vi "Scratchpad.vi"   [LabVIEW 2013]
uses:
  Classes/OSSP_Problem.lvclass
  Classes/GA.lvclass
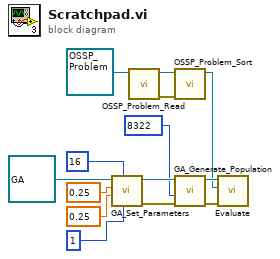
[diagram p0: block diagram]
diagram:
  n1 = call "GA_Set_Parameters.vi"("Population Size"=u8 1, "Dimension"=16, "Control 1Mutation Probability"=0.25, "Crossover Probability"=0.25, "GA in"=refnum<class "GA.lvclass"> refnum ("GA.lvclass")) -> ("error out"=w9:errorcluster, "GA out"=w10:refnum<class "GA.lvclass">)  [unwired: 5 in]
  n2 = call "OSSP_Problem_Read.vi"("OSSP_Problem.lvclass In"=refnum<class "OSSP_Problem.lvclass"> refnum ("OSSP_Problem.lvclass")) -> ("error out"=w12:errorcluster, "OSSP_Problem.lvclass Out"=w13:refnum<class "OSSP_Problem.lvclass">)  [unwired: 9 in]
  n3 = call "OSSP_Problem_Sort.vi"("error in (no error)"=w12, "OSSP_Problem.lvclass In"=w13) -> ("OSSP_Problem.lvclass Out"=w2:refnum<class "OSSP_Problem.lvclass">)  [unwired: 8 in, 1 out]
  n4 = call "GA_Generate_Population.vi"("error in (no error)"=w9, "seed"=8322, "GA in"=w10) -> ("error out"=w3:errorcluster, "GA out"=w4:refnum<class "GA.lvclass">)  [unwired: 7 in]
  n5 = call "Evaluate.vi"("error in (no error)"=w3, "OSSP_Problem.lvclass"=w2, "GA in"=w4) -> ()  [unwired: 6 in, 3 out]
